vi "Cal74100_update.vi"() -> ()   [LabVIEW 2014]
uses:
  <vilib>/Instr/_visa.llb/VISA Configure Serial Port (Instr).vi
panel:
  out "Info":string
  in  "Zero 3":string
  in  "Zero 2":string
  in  "Zero 1":string
  in  "Set":bool
  in  "Wavelength":string
  in  "Grat3":bool
  in  "Grat2":bool
  in  "Port2":bool
  in  "Port1":bool
  in  "Grat1":bool
  in  "CloseS":bool
  in  "OpenS":bool
  in  "Write":bool
  in  "Exit":bool
  in  "Read":bool
  in  "Label 3":string
  in  "Lines 3":string
  in  "Factor 3":string
  in  "Offset 3":string
  in  "Label 2":string
  in  "Lines 2":string
  in  "Factor 2":string
  in  "Offset 2":string
  in  "Offset 1":string
  in  "Factor 1":string
  in  "Lines 1":string
  in  "Label 1":string
  out "Current Grating":string
  out "State":string="ReadSettings"
  in  "Monochromator":refnum<visa-resource-name>="COM3"
  out "Next State":string="Wait"
  out "error":T1
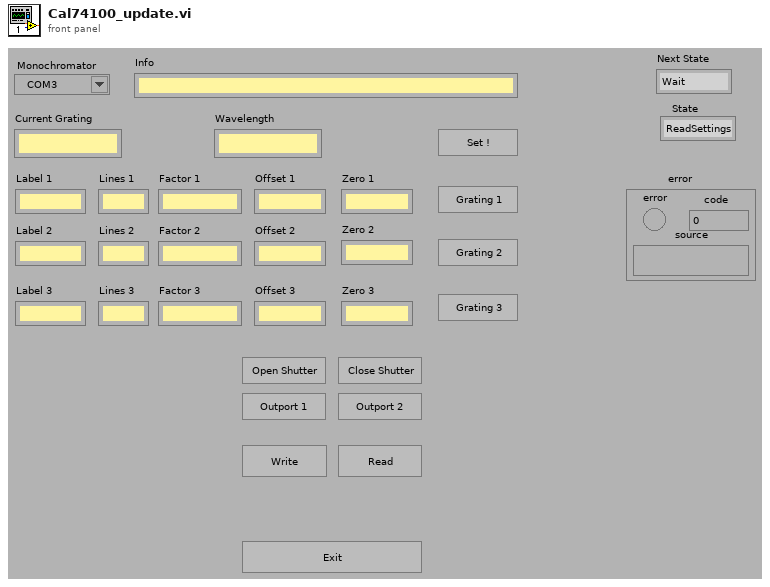
[diagram p1: front panel]
types:
  T1 = cluster{"error":bool, "code":i32, "source":string}
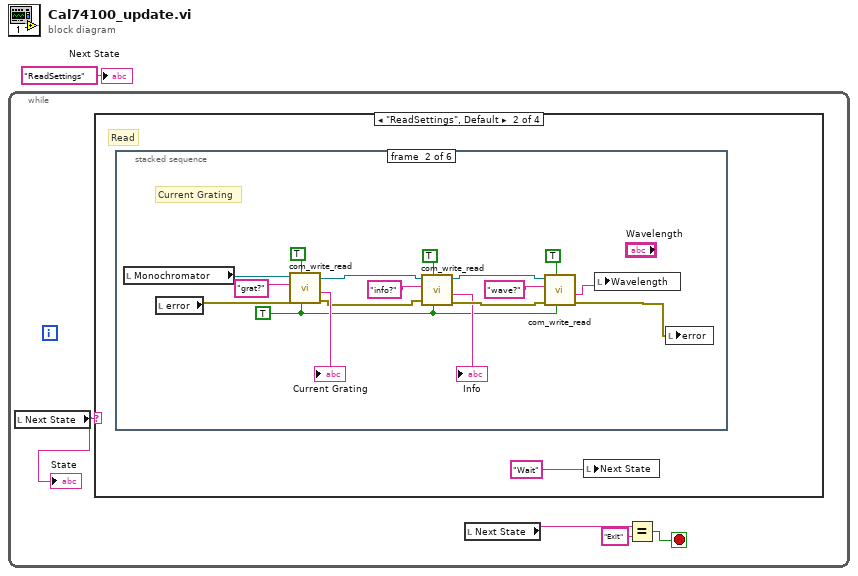
[diagram p0: block diagram]
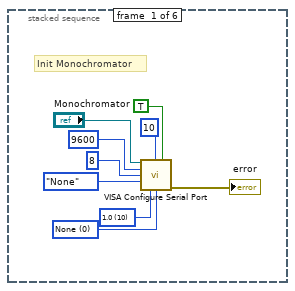
[diagram p3: hidden frame]
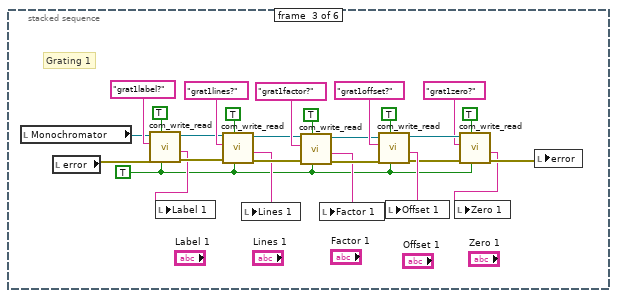
[diagram p4: hidden frame]
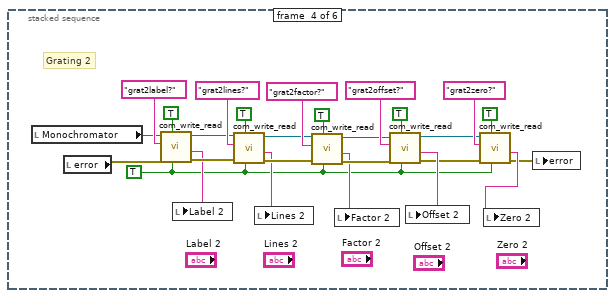
[diagram p5: hidden frame]
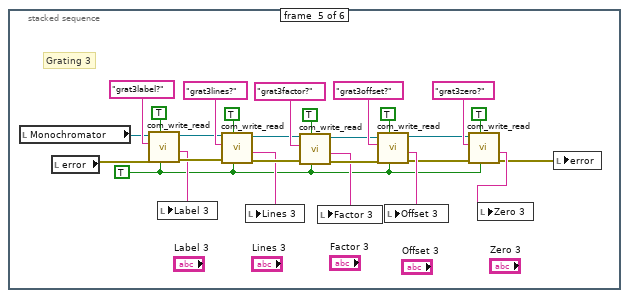
[diagram p6: hidden frame]
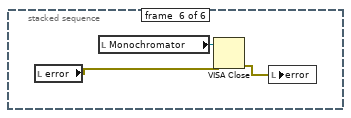
[diagram p7: hidden frame]
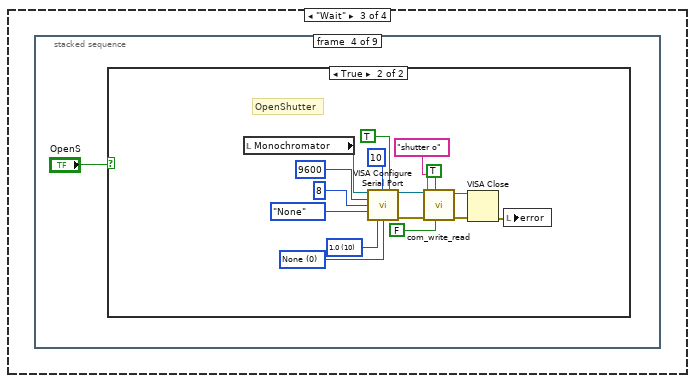
[diagram p8: hidden frame]
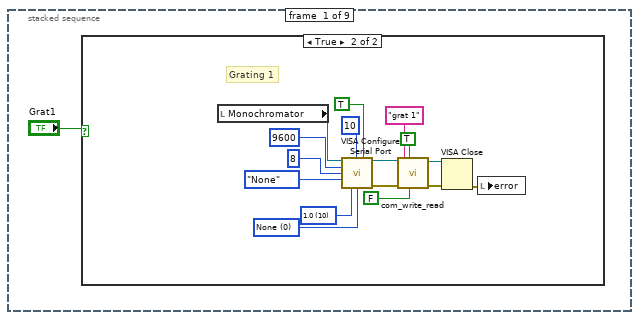
[diagram p9: hidden frame]
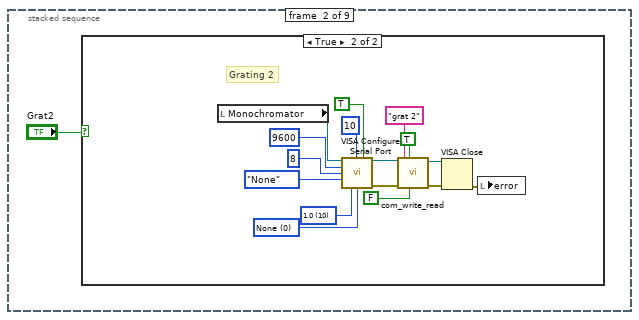
[diagram p11: hidden frame]
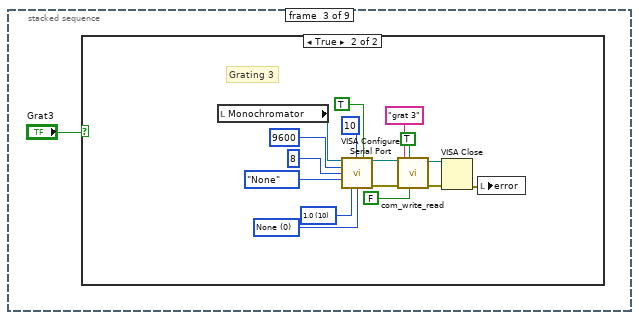
[diagram p13: hidden frame]
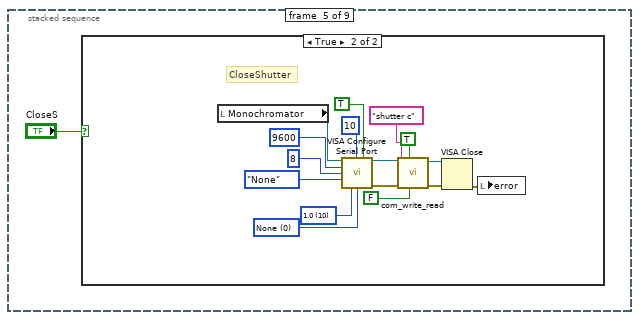
[diagram p16: hidden frame]
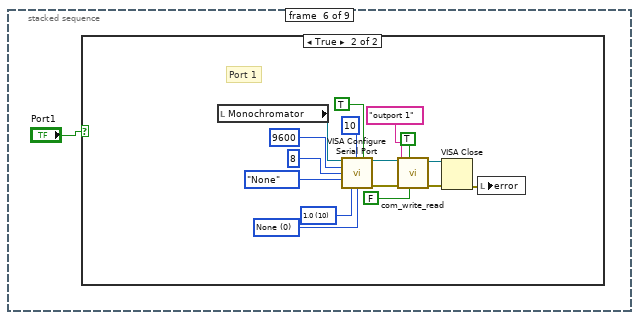
[diagram p18: hidden frame]
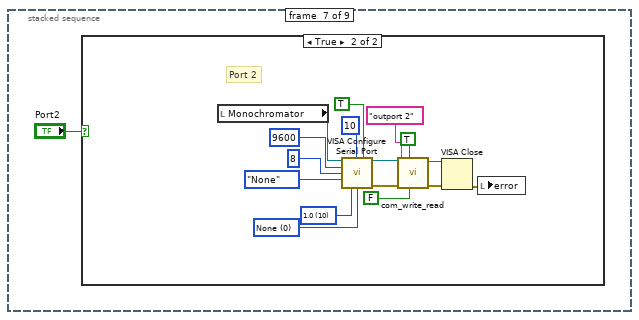
[diagram p20: hidden frame]
diagram:
  n1 = while {
    stop <- w4 stop-if-true
    n2 = local read "Next State"() -> (w2:string)
    "State" <- w2
    n3 = case shown="\"ReadSettings\", Default" w2 {
      frame "Exit" {
      }
      frame "ReadSettings", Default {
        # "Read"
        n4 = stacked-sequence {
          frame #0 {
            w13 = u16 0 items=["None", "XON/XOFF", "RTS/CTS", "XON/XOFF & RTS/CTS", "DTR/DSR", "XON/XOFF & DTR/DSR"] ("flow control (0:none)")
            w12 = u16 10 items=["1.0"=10, "1.5"=15, "2.0"=20] ("stop bits (10: 1 bit)")
            # "Init Monochromator"
            n5 = call-poly "VISA Configure Serial Port"("VISA resource name"="Monochromator", "termination char\n(0xA = '\\n' = LF)"=u8 10 ("termination char\n(0xA = '\\n' = LF)"), "Enable Termination\nChar (T)"=TRUE, "baud rate (9600)"=u32 9600, "data bits (8)"=u16 8, "parity (0:none)"=enum16{"None", "Odd", "Even", "Mark", "Space"}."None", "stop bits (10: 1 bit)"=w12, "flow control (0:none)"=w13) -> ("error out"=→"error":errorcluster)  [unwired: 6 in, 1 out]
          }
          frame #1 {
            w16 = TRUE ("2 nd Query?")
            # "Current Grating"
            n6 = local read "Monochromator"() -> (w29:refnum<visa-resource-name>)
            n7 = local read "error"() -> (w30:T1)
            n8 = call "com_write_read.vi"("2 nd Query?"=w16, "Query?"=TRUE, "error in"=w30, "Command"="grat?" ("write buffer"), "VISA handle in"=w29) -> ("error out"=w21:errorcluster, "2nd Response"=→"Current Grating":string, "VISA handle out"=w20:refnum<visa-resource-name>)  [unwired: 1 in, 2 out]
            n9 = call "com_write_read.vi"("2 nd Query?"=w16, "Query?"=TRUE, "error in"=w21, "Command"="info?" ("write buffer"), "VISA handle in"=w20) -> ("error out"=w18:errorcluster, "2nd Response"=→"Info":string, "VISA handle out"=w19:refnum<visa-resource-name>)  [unwired: 1 in, 2 out]
            n10 = call "com_write_read.vi"("2 nd Query?"=w16, "Query?"=TRUE, "error in"=w18, "Command"="wave?" ("write buffer"), "VISA handle in"=w19) -> ("error out"=w26:errorcluster, "2nd Response"=w24:string)  [unwired: 1 in, 3 out]
            n11 = local write "Wavelength"(w24) -> ()
            n12 = local write "error"(w26) -> ()
          }
          frame #2 {
            w33 = TRUE ("2 nd Query?")
            # "Grating 1"
            n13 = local read "Monochromator"() -> (w56:refnum<visa-resource-name>)
            n14 = local read "error"() -> (w57:T1)
            n15 = call "com_write_read.vi"("2 nd Query?"=w33, "Query?"=TRUE, "error in"=w57, "Command"="grat1label?" ("write buffer"), "VISA handle in"=w56) -> ("error out"=w46:errorcluster, "2nd Response"=w43:string, "VISA handle out"=w49:refnum<visa-resource-name>)  [unwired: 1 in, 2 out]
            n16 = local write "Label 1"(w43) -> ()
            n17 = call "com_write_read.vi"("2 nd Query?"=w33, "Query?"=TRUE, "error in"=w46, "Command"="grat1lines?" ("write buffer"), "VISA handle in"=w49) -> ("error out"=w45:errorcluster, "2nd Response"=w42:string, "VISA handle out"=w48:refnum<visa-resource-name>)  [unwired: 1 in, 2 out]
            n18 = local write "Lines 1"(w42) -> ()
            n19 = call "com_write_read.vi"("2 nd Query?"=w33, "Query?"=TRUE, "error in"=w45, "Command"="grat1factor?" ("write buffer"), "VISA handle in"=w48) -> ("error out"=w44:errorcluster, "2nd Response"=w41:string, "VISA handle out"=w47:refnum<visa-resource-name>)  [unwired: 1 in, 2 out]
            n20 = local write "Factor 1"(w41) -> ()
            n21 = call "com_write_read.vi"("2 nd Query?"=w33, "Query?"=TRUE, "error in"=w44, "Command"="grat1offset?" ("write buffer"), "VISA handle in"=w47) -> ("error out"=w37:errorcluster, "2nd Response"=w40:string, "VISA handle out"=w38:refnum<visa-resource-name>)  [unwired: 1 in, 2 out]
            n22 = local write "Offset 1"(w40) -> ()
            n23 = call "com_write_read.vi"("2 nd Query?"=w33, "Query?"=TRUE, "error in"=w37, "Command"="grat1zero?" ("write buffer"), "VISA handle in"=w38) -> ("error out"=w36:errorcluster, "2nd Response"=w35:string)  [unwired: 1 in, 3 out]
            n24 = local write "Zero 1"(w35) -> ()
            n25 = local write "error"(w36) -> ()
          }
          frame #3 {
            w60 = TRUE ("2 nd Query?")
            # "Grating 2"
            n26 = local read "Monochromator"() -> (w83:refnum<visa-resource-name>)
            n27 = local read "error"() -> (w84:T1)
            n28 = call "com_write_read.vi"("2 nd Query?"=w60, "Query?"=TRUE, "error in"=w84, "Command"="grat2label?" ("write buffer"), "VISA handle in"=w83) -> ("error out"=w73:errorcluster, "2nd Response"=w70:string, "VISA handle out"=w76:refnum<visa-resource-name>)  [unwired: 1 in, 2 out]
            n29 = local write "Label 2"(w70) -> ()
            n30 = call "com_write_read.vi"("2 nd Query?"=w60, "Query?"=TRUE, "error in"=w73, "Command"="grat2lines?" ("write buffer"), "VISA handle in"=w76) -> ("error out"=w72:errorcluster, "2nd Response"=w69:string, "VISA handle out"=w75:refnum<visa-resource-name>)  [unwired: 1 in, 2 out]
            n31 = local write "Lines 2"(w69) -> ()
            n32 = call "com_write_read.vi"("2 nd Query?"=w60, "Query?"=TRUE, "error in"=w72, "Command"="grat2factor?" ("write buffer"), "VISA handle in"=w75) -> ("error out"=w71:errorcluster, "2nd Response"=w68:string, "VISA handle out"=w74:refnum<visa-resource-name>)  [unwired: 1 in, 2 out]
            n33 = local write "Factor 2"(w68) -> ()
            n34 = call "com_write_read.vi"("2 nd Query?"=w60, "Query?"=TRUE, "error in"=w71, "Command"="grat2offset?" ("write buffer"), "VISA handle in"=w74) -> ("error out"=w63:errorcluster, "2nd Response"=w67:string, "VISA handle out"=w64:refnum<visa-resource-name>)  [unwired: 1 in, 2 out]
            n35 = local write "Offset 2"(w67) -> ()
            n36 = call "com_write_read.vi"("2 nd Query?"=w60, "Query?"=TRUE, "error in"=w63, "Command"="grat2zero?" ("write buffer"), "VISA handle in"=w64) -> ("error out"=w61:errorcluster, "2nd Response"=w62:string)  [unwired: 1 in, 3 out]
            n37 = local write "Zero 2"(w62) -> ()
            n38 = local write "error"(w61) -> ()
          }
          frame #4 {
            w87 = TRUE ("2 nd Query?")
            # "Grating 3"
            n39 = local read "Monochromator"() -> (w110:refnum<visa-resource-name>)
            n40 = local read "error"() -> (w111:T1)
            n41 = call "com_write_read.vi"("2 nd Query?"=w87, "Query?"=TRUE, "error in"=w111, "Command"="grat3label?" ("write buffer"), "VISA handle in"=w110) -> ("error out"=w100:errorcluster, "2nd Response"=w97:string, "VISA handle out"=w103:refnum<visa-resource-name>)  [unwired: 1 in, 2 out]
            n42 = local write "Label 3"(w97) -> ()
            n43 = call "com_write_read.vi"("2 nd Query?"=w87, "Query?"=TRUE, "error in"=w100, "Command"="grat3lines?" ("write buffer"), "VISA handle in"=w103) -> ("error out"=w99:errorcluster, "2nd Response"=w96:string, "VISA handle out"=w102:refnum<visa-resource-name>)  [unwired: 1 in, 2 out]
            n44 = local write "Lines 3"(w96) -> ()
            n45 = call "com_write_read.vi"("2 nd Query?"=w87, "Query?"=TRUE, "error in"=w99, "Command"="grat3factor?" ("write buffer"), "VISA handle in"=w102) -> ("error out"=w98:errorcluster, "2nd Response"=w95:string, "VISA handle out"=w101:refnum<visa-resource-name>)  [unwired: 1 in, 2 out]
            n46 = local write "Factor 3"(w95) -> ()
            n47 = call "com_write_read.vi"("2 nd Query?"=w87, "Query?"=TRUE, "error in"=w98, "Command"="grat3offset?" ("write buffer"), "VISA handle in"=w101) -> ("error out"=w90:errorcluster, "2nd Response"=w94:string, "VISA handle out"=w91:refnum<visa-resource-name>)  [unwired: 1 in, 2 out]
            n48 = local write "Offset 3"(w94) -> ()
            n49 = call "com_write_read.vi"("2 nd Query?"=w87, "Query?"=TRUE, "error in"=w90, "Command"="grat3zero?" ("write buffer"), "VISA handle in"=w91) -> ("error out"=w88:errorcluster, "2nd Response"=w89:string)  [unwired: 1 in, 3 out]
            n50 = local write "Zero 3"(w89) -> ()
            n51 = local write "error"(w88) -> ()
          }
          frame #5 {
            n52 = local read "error"() -> (w114:T1)
            n53 = local read "Monochromator"() -> (w116:refnum<visa-resource-name>)
            n54 = VISA Close(VISA resource name=w116, error in (no error)=w114) -> (error out=w115:errorcluster)
            n55 = local write "error"(w115) -> ()
          }
        }
        n56 = local write "Next State"("Wait") -> ()
      }
      frame "Wait" {
        n57 = stacked-sequence {
          frame #0 {
            n58 = case shown="True" "Grat1" {
              frame False {
              }
              frame True {
                w121 = u16 0 items=["None", "XON/XOFF", "RTS/CTS", "XON/XOFF & RTS/CTS", "DTR/DSR", "XON/XOFF & DTR/DSR"] ("flow control (0:none)")
                w122 = u16 10 items=["1.0"=10, "1.5"=15, "2.0"=20] ("stop bits (10: 1 bit)")
                # "Grating 1"
                n59 = local read "Monochromator"() -> (w126:refnum<visa-resource-name>)
                n60 = call-poly "VISA Configure Serial Port"("VISA resource name"=w126, "termination char\n(0xA = '\\n' = LF)"=u8 10 ("termination char\n(0xA = '\\n' = LF)"), "Enable Termination\nChar (T)"=TRUE, "baud rate (9600)"=u32 9600, "data bits (8)"=u16 8, "parity (0:none)"=enum16{"None", "Odd", "Even", "Mark", "Space"}."None", "stop bits (10: 1 bit)"=w122, "flow control (0:none)"=w121) -> ("VISA resource name out"=w131:refnum<visa-resource-name>, "error out"=w130:errorcluster)  [unwired: 6 in]
                n61 = call "com_write_read.vi"("2 nd Query?"=FALSE, "Query?"=TRUE, "error in"=w130, "Command"="grat 1" ("write buffer"), "VISA handle in"=w131) -> ("error out"=w133:errorcluster, "VISA handle out"=w132:refnum<visa-resource-name>)  [unwired: 1 in, 3 out]
                n62 = VISA Close(VISA resource name=w132, error in (no error)=w133) -> (error out=w127:errorcluster)
                n63 = local write "error"(w127) -> ()
              }
            }
          }
          frame #1 {
            n64 = case shown="True" "Grat2" {
              frame False {
              }
              frame True {
                w138 = u16 0 items=["None", "XON/XOFF", "RTS/CTS", "XON/XOFF & RTS/CTS", "DTR/DSR", "XON/XOFF & DTR/DSR"] ("flow control (0:none)")
                w139 = u16 10 items=["1.0"=10, "1.5"=15, "2.0"=20] ("stop bits (10: 1 bit)")
                # "Grating 2"
                n65 = local read "Monochromator"() -> (w143:refnum<visa-resource-name>)
                n66 = call-poly "VISA Configure Serial Port"("VISA resource name"=w143, "termination char\n(0xA = '\\n' = LF)"=u8 10 ("termination char\n(0xA = '\\n' = LF)"), "Enable Termination\nChar (T)"=TRUE, "baud rate (9600)"=u32 9600, "data bits (8)"=u16 8, "parity (0:none)"=enum16{"None", "Odd", "Even", "Mark", "Space"}."None", "stop bits (10: 1 bit)"=w139, "flow control (0:none)"=w138) -> ("VISA resource name out"=w148:refnum<visa-resource-name>, "error out"=w147:errorcluster)  [unwired: 6 in]
                n67 = call "com_write_read.vi"("2 nd Query?"=FALSE, "Query?"=TRUE, "error in"=w147, "Command"="grat 2" ("write buffer"), "VISA handle in"=w148) -> ("error out"=w150:errorcluster, "VISA handle out"=w149:refnum<visa-resource-name>)  [unwired: 1 in, 3 out]
                n68 = VISA Close(VISA resource name=w149, error in (no error)=w150) -> (error out=w144:errorcluster)
                n69 = local write "error"(w144) -> ()
              }
            }
          }
          frame #2 {
            n70 = case shown="True" "Grat3" {
              frame False {
              }
              frame True {
                w155 = u16 0 items=["None", "XON/XOFF", "RTS/CTS", "XON/XOFF & RTS/CTS", "DTR/DSR", "XON/XOFF & DTR/DSR"] ("flow control (0:none)")
                w156 = u16 10 items=["1.0"=10, "1.5"=15, "2.0"=20] ("stop bits (10: 1 bit)")
                # "Grating 3"
                n71 = local read "Monochromator"() -> (w160:refnum<visa-resource-name>)
                n72 = call-poly "VISA Configure Serial Port"("VISA resource name"=w160, "termination char\n(0xA = '\\n' = LF)"=u8 10 ("termination char\n(0xA = '\\n' = LF)"), "Enable Termination\nChar (T)"=TRUE, "baud rate (9600)"=u32 9600, "data bits (8)"=u16 8, "parity (0:none)"=enum16{"None", "Odd", "Even", "Mark", "Space"}."None", "stop bits (10: 1 bit)"=w156, "flow control (0:none)"=w155) -> ("VISA resource name out"=w165:refnum<visa-resource-name>, "error out"=w164:errorcluster)  [unwired: 6 in]
                n73 = call "com_write_read.vi"("2 nd Query?"=FALSE, "Query?"=TRUE, "error in"=w164, "Command"="grat 3" ("write buffer"), "VISA handle in"=w165) -> ("error out"=w167:errorcluster, "VISA handle out"=w166:refnum<visa-resource-name>)  [unwired: 1 in, 3 out]
                n74 = VISA Close(VISA resource name=w166, error in (no error)=w167) -> (error out=w161:errorcluster)
                n75 = local write "error"(w161) -> ()
              }
            }
          }
          frame #3 {
            n76 = case shown="True" "OpenS" {
              frame False {
              }
              frame True {
                w172 = u16 0 items=["None", "XON/XOFF", "RTS/CTS", "XON/XOFF & RTS/CTS", "DTR/DSR", "XON/XOFF & DTR/DSR"] ("flow control (0:none)")
                w173 = u16 10 items=["1.0"=10, "1.5"=15, "2.0"=20] ("stop bits (10: 1 bit)")
                # "OpenShutter"
                n77 = local read "Monochromator"() -> (w177:refnum<visa-resource-name>)
                n78 = call-poly "VISA Configure Serial Port"("VISA resource name"=w177, "termination char\n(0xA = '\\n' = LF)"=u8 10 ("termination char\n(0xA = '\\n' = LF)"), "Enable Termination\nChar (T)"=TRUE, "baud rate (9600)"=u32 9600, "data bits (8)"=u16 8, "parity (0:none)"=enum16{"None", "Odd", "Even", "Mark", "Space"}."None", "stop bits (10: 1 bit)"=w173, "flow control (0:none)"=w172) -> ("VISA resource name out"=w182:refnum<visa-resource-name>, "error out"=w181:errorcluster)  [unwired: 6 in]
                n79 = call "com_write_read.vi"("2 nd Query?"=FALSE, "Query?"=TRUE, "error in"=w181, "Command"="shutter o" ("write buffer"), "VISA handle in"=w182) -> ("error out"=w184:errorcluster, "VISA handle out"=w183:refnum<visa-resource-name>)  [unwired: 1 in, 3 out]
                n80 = VISA Close(VISA resource name=w183, error in (no error)=w184) -> (error out=w178:errorcluster)
                n81 = local write "error"(w178) -> ()
              }
            }
          }
          frame #4 {
            n82 = case shown="True" "CloseS" {
              frame False {
              }
              frame True {
                w189 = u16 0 items=["None", "XON/XOFF", "RTS/CTS", "XON/XOFF & RTS/CTS", "DTR/DSR", "XON/XOFF & DTR/DSR"] ("flow control (0:none)")
                w190 = u16 10 items=["1.0"=10, "1.5"=15, "2.0"=20] ("stop bits (10: 1 bit)")
                # "CloseShutter"
                n83 = local read "Monochromator"() -> (w194:refnum<visa-resource-name>)
                n84 = call-poly "VISA Configure Serial Port"("VISA resource name"=w194, "termination char\n(0xA = '\\n' = LF)"=u8 10 ("termination char\n(0xA = '\\n' = LF)"), "Enable Termination\nChar (T)"=TRUE, "baud rate (9600)"=u32 9600, "data bits (8)"=u16 8, "parity (0:none)"=enum16{"None", "Odd", "Even", "Mark", "Space"}."None", "stop bits (10: 1 bit)"=w190, "flow control (0:none)"=w189) -> ("VISA resource name out"=w199:refnum<visa-resource-name>, "error out"=w198:errorcluster)  [unwired: 6 in]
                n85 = call "com_write_read.vi"("2 nd Query?"=FALSE, "Query?"=TRUE, "error in"=w198, "Command"="shutter c" ("write buffer"), "VISA handle in"=w199) -> ("error out"=w201:errorcluster, "VISA handle out"=w200:refnum<visa-resource-name>)  [unwired: 1 in, 3 out]
                n86 = VISA Close(VISA resource name=w200, error in (no error)=w201) -> (error out=w195:errorcluster)
                n87 = local write "error"(w195) -> ()
              }
            }
          }
          frame #5 {
            n88 = case shown="True" "Port1" {
              frame False {
              }
              frame True {
                w206 = u16 0 items=["None", "XON/XOFF", "RTS/CTS", "XON/XOFF & RTS/CTS", "DTR/DSR", "XON/XOFF & DTR/DSR"] ("flow control (0:none)")
                w207 = u16 10 items=["1.0"=10, "1.5"=15, "2.0"=20] ("stop bits (10: 1 bit)")
                # "Port 1"
                n89 = local read "Monochromator"() -> (w211:refnum<visa-resource-name>)
                n90 = call-poly "VISA Configure Serial Port"("VISA resource name"=w211, "termination char\n(0xA = '\\n' = LF)"=u8 10 ("termination char\n(0xA = '\\n' = LF)"), "Enable Termination\nChar (T)"=TRUE, "baud rate (9600)"=u32 9600, "data bits (8)"=u16 8, "parity (0:none)"=enum16{"None", "Odd", "Even", "Mark", "Space"}."None", "stop bits (10: 1 bit)"=w207, "flow control (0:none)"=w206) -> ("VISA resource name out"=w216:refnum<visa-resource-name>, "error out"=w215:errorcluster)  [unwired: 6 in]
                n91 = call "com_write_read.vi"("2 nd Query?"=FALSE, "Query?"=TRUE, "error in"=w215, "Command"="outport 1" ("write buffer"), "VISA handle in"=w216) -> ("error out"=w218:errorcluster, "VISA handle out"=w217:refnum<visa-resource-name>)  [unwired: 1 in, 3 out]
                n92 = VISA Close(VISA resource name=w217, error in (no error)=w218) -> (error out=w212:errorcluster)
                n93 = local write "error"(w212) -> ()
              }
            }
          }
          frame #6 {
            n94 = case shown="True" "Port2" {
              frame False {
              }
              frame True {
                w223 = u16 0 items=["None", "XON/XOFF", "RTS/CTS", "XON/XOFF & RTS/CTS", "DTR/DSR", "XON/XOFF & DTR/DSR"] ("flow control (0:none)")
                w224 = u16 10 items=["1.0"=10, "1.5"=15, "2.0"=20] ("stop bits (10: 1 bit)")
                # "Port 2"
                n95 = local read "Monochromator"() -> (w228:refnum<visa-resource-name>)
                n96 = call-poly "VISA Configure Serial Port"("VISA resource name"=w228, "termination char\n(0xA = '\\n' = LF)"=u8 10 ("termination char\n(0xA = '\\n' = LF)"), "Enable Termination\nChar (T)"=TRUE, "baud rate (9600)"=u32 9600, "data bits (8)"=u16 8, "parity (0:none)"=enum16{"None", "Odd", "Even", "Mark", "Space"}."None", "stop bits (10: 1 bit)"=w224, "flow control (0:none)"=w223) -> ("VISA resource name out"=w233:refnum<visa-resource-name>, "error out"=w232:errorcluster)  [unwired: 6 in]
                n97 = call "com_write_read.vi"("2 nd Query?"=FALSE, "Query?"=TRUE, "error in"=w232, "Command"="outport 2" ("write buffer"), "VISA handle in"=w233) -> ("error out"=w235:errorcluster, "VISA handle out"=w234:refnum<visa-resource-name>)  [unwired: 1 in, 3 out]
                n98 = VISA Close(VISA resource name=w234, error in (no error)=w235) -> (error out=w229:errorcluster)
                n99 = local write "error"(w229) -> ()
              }
            }
          }
          frame #7 {
            n100 = case shown="True" "Set" {
              frame False {
              }
              frame True {
                w245 = u16 0 items=["None", "XON/XOFF", "RTS/CTS", "XON/XOFF & RTS/CTS", "DTR/DSR", "XON/XOFF & DTR/DSR"] ("flow control (0:none)")
                w246 = u16 10 items=["1.0"=10, "1.5"=15, "2.0"=20] ("stop bits (10: 1 bit)")
                # "Set Wavelength"
                n101 = local read "Monochromator"() -> (w250:refnum<visa-resource-name>)
                n102 = call-poly "VISA Configure Serial Port"("VISA resource name"=w250, "termination char\n(0xA = '\\n' = LF)"=u8 10 ("termination char\n(0xA = '\\n' = LF)"), "Enable Termination\nChar (T)"=TRUE, "baud rate (9600)"=u32 9600, "data bits (8)"=u16 8, "parity (0:none)"=enum16{"None", "Odd", "Even", "Mark", "Space"}."None", "stop bits (10: 1 bit)"=w246, "flow control (0:none)"=w245) -> ("VISA resource name out"=w254:refnum<visa-resource-name>, "error out"=w253:errorcluster)  [unwired: 6 in]
                n103 = local read "Wavelength"() -> (w239:string)
                n104 = String Subset(string=w239, length (rest)=8 ("length (rest)")) -> (substring=w242:string)  [unwired: 1 in]
                n105 = Concatenate Strings("gowave " ("write buffer"), w242) -> (w238:string)
                n106 = call "com_write_read.vi"("2 nd Query?"=FALSE, "Query?"=TRUE, "error in"=w253, "Command"=w238, "VISA handle in"=w254) -> ("error out"=w256:errorcluster, "VISA handle out"=w255:refnum<visa-resource-name>)  [unwired: 1 in, 3 out]
                n107 = VISA Close(VISA resource name=w255, error in (no error)=w256) -> (error out=w251:errorcluster)
                n108 = local write "error"(w251) -> ()
              }
            }
          }
          frame #8 {
            n109 = local read "Next State"() -> (w258:string)
            n110 = Select(t="Write", s="Write", f=w258) -> (s? t:f=w260:string)
            n111 = Select(t="Read", s="Read", f=w260) -> (s? t:f=w262:string)
            n112 = Select(t="Exit", s="Exit", f=w262) -> (s? t:f=w263:string)
            n113 = local write "Next State"(w263) -> ()
          }
        }
      }
      frame "Write" {
        # "Write"
        n114 = stacked-sequence {
          frame #0 {
            w274 = u16 0 items=["None", "XON/XOFF", "RTS/CTS", "XON/XOFF & RTS/CTS", "DTR/DSR", "XON/XOFF & DTR/DSR"] ("flow control (0:none)")
            w273 = u16 10 items=["1.0"=10, "1.5"=15, "2.0"=20] ("stop bits (10: 1 bit)")
            # "Init Monochromator"
            n115 = local read "Monochromator"() -> (w268:refnum<visa-resource-name>)
            n116 = call-poly "VISA Configure Serial Port"("VISA resource name"=w268, "termination char\n(0xA = '\\n' = LF)"=u8 10 ("termination char\n(0xA = '\\n' = LF)"), "Enable Termination\nChar (T)"=TRUE, "baud rate (9600)"=u32 9600, "data bits (8)"=u16 8, "parity (0:none)"=enum16{"None", "Odd", "Even", "Mark", "Space"}."None", "stop bits (10: 1 bit)"=w273, "flow control (0:none)"=w274) -> ("error out"=w269:errorcluster)  [unwired: 6 in, 1 out]
            n117 = local write "error"(w269) -> ()
          }
          frame #1 {
            # "Grating 1"
            n118 = local read "Monochromator"() -> (w307:refnum<visa-resource-name>)
            n119 = local read "Label 1"() -> (w293:string)
            n120 = local read "error"() -> (w308:T1)
            n121 = String Subset(string=w293, length (rest)=8 ("length (rest)")) -> (substring=w296:string)  [unwired: 1 in]
            n122 = Concatenate Strings("grat1label " ("write buffer"), w296) -> (w280:string)
            n123 = local read "Offset 1"() -> (w292:string)
            n124 = call "com_write_read.vi"("Query?"=TRUE, "error in"=w308, "Command"=w280, "VISA handle in"=w307) -> ("error out"=w300:errorcluster, "VISA handle out"=w303:refnum<visa-resource-name>)  [unwired: 2 in, 3 out]
            n125 = String Subset(string=w292, length (rest)=8 ("length (rest)")) -> (substring=w289:string)  [unwired: 1 in]
            n126 = Concatenate Strings("grat1offset " ("write buffer"), w289) -> (w279:string)
            n127 = local read "Lines 1"() -> (w288:string)
            n128 = call "com_write_read.vi"("Query?"=TRUE, "error in"=w300, "Command"=w279, "VISA handle in"=w303) -> ("error out"=w299:errorcluster, "VISA handle out"=w302:refnum<visa-resource-name>)  [unwired: 2 in, 3 out]
            n129 = String Subset(string=w288, length (rest)=8 ("length (rest)")) -> (substring=w285:string)  [unwired: 1 in]
            n130 = Concatenate Strings("grat1lines " ("write buffer"), w285) -> (w278:string)
            n131 = local read "Factor 1"() -> (w284:string)
            n132 = call "com_write_read.vi"("Query?"=TRUE, "error in"=w299, "Command"=w278, "VISA handle in"=w302) -> ("error out"=w298:errorcluster, "VISA handle out"=w301:refnum<visa-resource-name>)  [unwired: 2 in, 3 out]
            n133 = String Subset(string=w284, length (rest)=8 ("length (rest)")) -> (substring=w281:string)  [unwired: 1 in]
            n134 = Concatenate Strings("grat1factor " ("write buffer"), w281) -> (w277:string)
            n135 = call "com_write_read.vi"("Query?"=TRUE, "error in"=w298, "Command"=w277, "VISA handle in"=w301) -> ("error out"=w297:errorcluster)  [unwired: 2 in, 4 out]
            n136 = local write "error"(w297) -> ()
          }
          frame #2 {
            # "Grating 2"
            n137 = local read "Monochromator"() -> (w340:refnum<visa-resource-name>)
            n138 = local read "Label 2"() -> (w326:string)
            n139 = local read "error"() -> (w341:T1)
            n140 = String Subset(string=w326, length (rest)=8 ("length (rest)")) -> (substring=w329:string)  [unwired: 1 in]
            n141 = Concatenate Strings("grat2label " ("write buffer"), w329) -> (w313:string)
            n142 = local read "Offset 2"() -> (w325:string)
            n143 = call "com_write_read.vi"("Query?"=TRUE, "error in"=w341, "Command"=w313, "VISA handle in"=w340) -> ("error out"=w333:errorcluster, "VISA handle out"=w336:refnum<visa-resource-name>)  [unwired: 2 in, 3 out]
            n144 = String Subset(string=w325, length (rest)=8 ("length (rest)")) -> (substring=w322:string)  [unwired: 1 in]
            n145 = Concatenate Strings("grat2offset " ("write buffer"), w322) -> (w312:string)
            n146 = local read "Lines 2"() -> (w321:string)
            n147 = call "com_write_read.vi"("Query?"=TRUE, "error in"=w333, "Command"=w312, "VISA handle in"=w336) -> ("error out"=w332:errorcluster, "VISA handle out"=w335:refnum<visa-resource-name>)  [unwired: 2 in, 3 out]
            n148 = String Subset(string=w321, length (rest)=8 ("length (rest)")) -> (substring=w318:string)  [unwired: 1 in]
            n149 = Concatenate Strings("grat2lines " ("write buffer"), w318) -> (w311:string)
            n150 = local read "Factor 2"() -> (w317:string)
            n151 = call "com_write_read.vi"("Query?"=TRUE, "error in"=w332, "Command"=w311, "VISA handle in"=w335) -> ("error out"=w331:errorcluster, "VISA handle out"=w334:refnum<visa-resource-name>)  [unwired: 2 in, 3 out]
            n152 = String Subset(string=w317, length (rest)=8 ("length (rest)")) -> (substring=w314:string)  [unwired: 1 in]
            n153 = Concatenate Strings("grat2factor " ("write buffer"), w314) -> (w310:string)
            n154 = call "com_write_read.vi"("Query?"=TRUE, "error in"=w331, "Command"=w310, "VISA handle in"=w334) -> ("error out"=w330:errorcluster)  [unwired: 2 in, 4 out]
            n155 = local write "error"(w330) -> ()
          }
          frame #3 {
            # "Grating 3"
            n156 = local read "Monochromator"() -> (w373:refnum<visa-resource-name>)
            n157 = local read "Label 3"() -> (w359:string)
            n158 = local read "error"() -> (w374:T1)
            n159 = String Subset(string=w359, length (rest)=8 ("length (rest)")) -> (substring=w362:string)  [unwired: 1 in]
            n160 = Concatenate Strings("grat3label " ("write buffer"), w362) -> (w346:string)
            n161 = local read "Offset 3"() -> (w358:string)
            n162 = call "com_write_read.vi"("Query?"=TRUE, "error in"=w374, "Command"=w346, "VISA handle in"=w373) -> ("error out"=w366:errorcluster, "VISA handle out"=w369:refnum<visa-resource-name>)  [unwired: 2 in, 3 out]
            n163 = String Subset(string=w358, length (rest)=8 ("length (rest)")) -> (substring=w355:string)  [unwired: 1 in]
            n164 = Concatenate Strings("grat3offset " ("write buffer"), w355) -> (w345:string)
            n165 = local read "Lines 3"() -> (w354:string)
            n166 = call "com_write_read.vi"("Query?"=TRUE, "error in"=w366, "Command"=w345, "VISA handle in"=w369) -> ("error out"=w365:errorcluster, "VISA handle out"=w368:refnum<visa-resource-name>)  [unwired: 2 in, 3 out]
            n167 = String Subset(string=w354, length (rest)=8 ("length (rest)")) -> (substring=w351:string)  [unwired: 1 in]
            n168 = Concatenate Strings("grat3lines " ("write buffer"), w351) -> (w344:string)
            n169 = local read "Factor 3"() -> (w350:string)
            n170 = call "com_write_read.vi"("Query?"=TRUE, "error in"=w365, "Command"=w344, "VISA handle in"=w368) -> ("error out"=w364:errorcluster, "VISA handle out"=w367:refnum<visa-resource-name>)  [unwired: 2 in, 3 out]
            n171 = String Subset(string=w350, length (rest)=8 ("length (rest)")) -> (substring=w347:string)  [unwired: 1 in]
            n172 = Concatenate Strings("grat3factor " ("write buffer"), w347) -> (w343:string)
            n173 = call "com_write_read.vi"("Query?"=TRUE, "error in"=w364, "Command"=w343, "VISA handle in"=w367) -> ("error out"=w363:errorcluster)  [unwired: 2 in, 4 out]
            n174 = local write "error"(w363) -> ()
          }
          frame #4 {
            # "Grating Zeros"
            n175 = local read "Monochromator"() -> (w398:refnum<visa-resource-name>)
            n176 = local read "Zero 1"() -> (w388:string)
            n177 = local read "error"() -> (w399:T1)
            n178 = String Subset(string=w388, length (rest)=8 ("length (rest)")) -> (substring=w391:string)  [unwired: 1 in]
            n179 = Concatenate Strings("grat1zero " ("write buffer"), w391) -> (w379:string)
            n180 = call "com_write_read.vi"("Query?"=TRUE, "error in"=w399, "Command"=w379, "VISA handle in"=w398) -> ("error out"=w393:errorcluster, "VISA handle out"=w395:refnum<visa-resource-name>)  [unwired: 2 in, 3 out]
            n181 = local read "Zero 2"() -> (w387:string)
            n182 = String Subset(string=w387, length (rest)=8 ("length (rest)")) -> (substring=w384:string)  [unwired: 1 in]
            n183 = Concatenate Strings("grat2zero " ("write buffer"), w384) -> (w378:string)
            n184 = local read "Zero 3"() -> (w383:string)
            n185 = call "com_write_read.vi"("Query?"=TRUE, "error in"=w393, "Command"=w378, "VISA handle in"=w395) -> ("error out"=w392:errorcluster, "VISA handle out"=w394:refnum<visa-resource-name>)  [unwired: 2 in, 3 out]
            n186 = String Subset(string=w383, length (rest)=8 ("length (rest)")) -> (substring=w380:string)  [unwired: 1 in]
            n187 = Concatenate Strings("grat3zero " ("write buffer"), w380) -> (w377:string)
            n188 = call "com_write_read.vi"("Query?"=TRUE, "error in"=w392, "Command"=w377, "VISA handle in"=w394) -> ("error out"=w376:errorcluster)  [unwired: 2 in, 4 out]
            n189 = local write "error"(w376) -> ()
          }
          frame #5 {
            n190 = local read "error"() -> (w401:T1)
            n191 = local read "Monochromator"() -> (w403:refnum<visa-resource-name>)
            n192 = VISA Close(VISA resource name=w403, error in (no error)=w401) -> (error out=w402:errorcluster)
            n193 = local write "error"(w402) -> ()
          }
        }
        n194 = local write "Next State"("Wait") -> ()
      }
    }
    n195 = local read "Next State"() -> (w5:string)
    n196 = Equal?(x=w5, y="Exit") -> (x = y?=w4:bool)
  }
  "Next State" <- "ReadSettings"
